vi "preamble.vi"(11 "Preamble Length (bits)":u32) -> (3 "Preamble":i32[](array[numeric]))   [LabVIEW 2012]
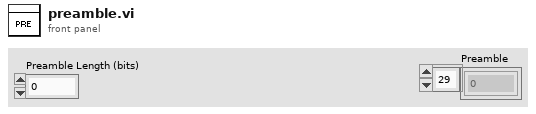
[diagram p1: front panel]
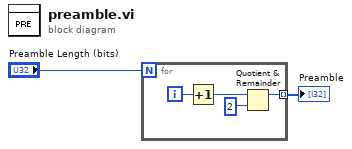
[diagram p0: block diagram]
diagram:
  n1 = for {
    N: "Preamble Length (bits)" -> [_]
    tunnel: [w3] -> w2 mode=indexing
    i -> [w5]
    n2 = Increment(x=w5) -> (x+1=w4:i32)
    n3 = Quotient & Remainder(x=w4, y=2) -> (x-y*floor(x/y)=w3:i32)  [unwired: 1 out]
  }
  "Preamble" <- w2
